vi "23384_Davis_Poku_Amankwa_Amankwa.DavisPoku.MNE1201.1.3_348251_94510281.vi"() -> ()   [LabVIEW 2018]
panel:
  out "R":dbl
  in  "R2":dbl
  in  "R1":dbl
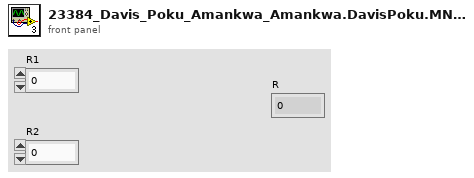
[diagram p1: front panel]
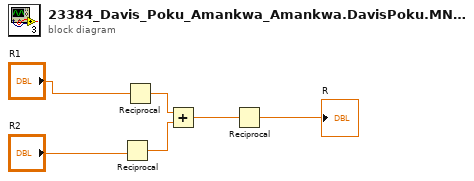
[diagram p0: block diagram]
diagram:
  n1 = Reciprocal(x="R2") -> (1/x=w4:dbl)
  n2 = Reciprocal(x="R1") -> (1/x=w3:dbl)
  n3 = Add(x=w3, y=w4) -> (x+y=w2:dbl)
  n4 = Reciprocal(x=w2) -> (1/x=→"R":dbl)
